vi "Read Image.vi"(8 "error in (no error)":errorcluster, 11 "Image Msg in":refnum<class "Image Msg.lvclass">) -> (0 "error out":errorcluster, 2 "Image":T1, 3 "Image Msg out":refnum<class "Image Msg.lvclass">)   [LabVIEW 2015, in "UI.lvlib" / "Image Msg.lvclass"]
uses:
  Image Msg.lvclass
  <vilib>/vision/Image Controls.llb/IMAQ Image.ctl
  Image Msg.lvclass/Image Msg.ctl
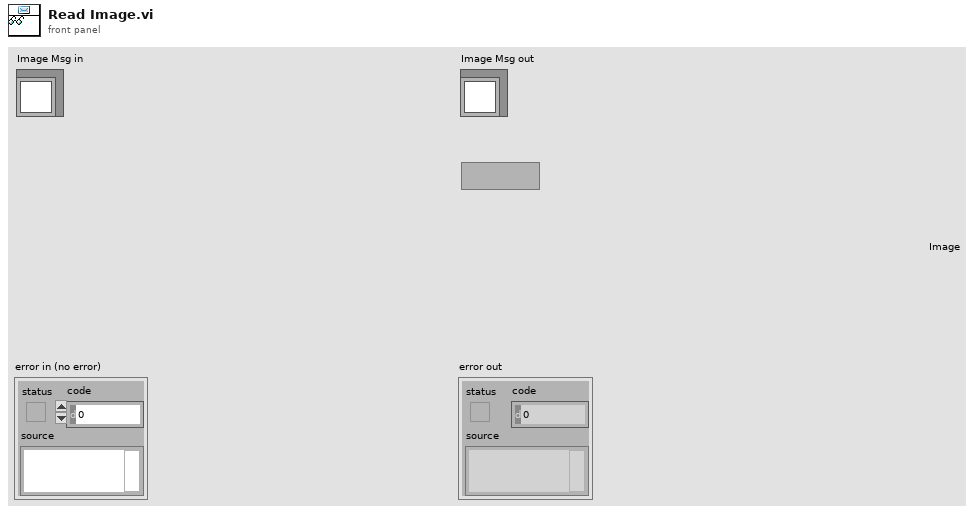
[diagram p1: front panel]
types:
  T1 = typedef "IMAQ Image.ctl" = refnum<image>
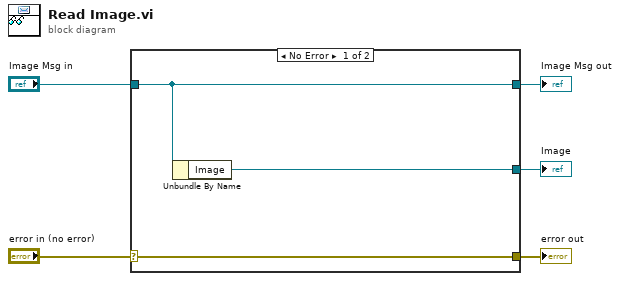
[diagram p0: block diagram]
diagram:
  n1 = case shown="No Error" "error in (no error)" {
    selector: "error in (no error)" -> [w8 w9]
    tunnel: [w8 w9] -> w4
    tunnel: [w7 w10] -> w2
    tunnel: "Image Msg in" -> [w7 w10]
    tunnel: [w6 _] -> w1
    frame No Error {
      n2 = Unbundle By Name(w7) -> ("Image"=w6:T1)
    }
    frame Error {
    }
  }
  "error out" <- w4
  "Image Msg out" <- w2
  "Image" <- w1
